vi "TEST_ASIC_MAJnADDS.vi"(0 "Instrument VISA in":T1={"AWG VISA"="generadorpulsos", "Oscilloscope  VISA "="Oscilloscope", "Integration Board IP"="172.16.7.43", "connection ID"=refnum, "report out"=refnum, "report file path"=path "C:/Documents and Settings/CTA_LAB01/Desktop/L0_Asic/L0 Asic Test "}, 1 "threshold":i32[][](array[numeric]), 2 "Serial number":string="SN002", 5 "quantity":i32=3, 7 "Cycles Burst":i32=10000, 11 "error in":errorcluster={"status"=FALSE, "code"=0, "source"="VISA Write in Test2_3a_ASIC_fast.vi->test_sum_ASIC.vi"}, 12 "channel array":i32[](array[numeric])=[0, 1, 2, 3, 4, 5, 6], 13 "Voltages comprobation":dbl[](array[numeric])=[0.05, 0.8]) -> (4 "Instrument VISA out":T1={"AWG VISA"="", "Oscilloscope  VISA "="", "Integration Board IP"="", "connection ID"=refnum, "report out"=refnum, "report file path"=path "C:/Documents and Settings/CTA_LAB01/Desktop/L0_Asic/L0 Asic Test "}, 15 "error out":errorcluster)   [LabVIEW 2009]
uses:
  <vilib>/Utility/NIReport.llb/NI_report.lvclass
  <vilib>/Utility/NIReport.llb/HTML/NI_HTML.lvclass
  <instrlib>/Agilent 81150/Agilent 81150.lvlib
  <instrlib>/Agilent 8000 Series/Agilent 8000 Series.lvlib
panel:
  out "read buffer 4":string="V amptd(f2),1.074E+00,0,1.056E+00,1.087E+00,1.0690E+00,5.5E-03,9.4E+01,+ width(f2),2.90015E-09,0,2.90015E-09,2.95960E-09,2.925838E-09,1.2702E-11,9.4E+01,V amptd(1),5.5E-02,0,4.8E-02,6.7E-02,5.55E-02,3.5E-03,9.4E+01,+ width(f1),9.99999E+37,5,9.99999E+37,9.99999E+37,9.99999E+37,9.99999E+37,9.99999E+37,Time(f1-f2),6.26722E-09,0,6.20145E-09,6.35270E-09,6.264189E-09,3.2805E-11,9.4E+01\n"
  out "report file path":path=path "C:/Documents and Settings/CTA_LAB01/Desktop/L0_Asic/L0 Asic Test "
  out "Array":i32[](array[numeric])=[2, 3, 5]
  out "points quantity":dbl=94.0
  out "ouput data array":dbl[](array[numeric])=[0.75, 42.0, 0.0, 63.0, 1.0, 1.069, 0.0055, 2.925838e-09, 1.2702e-11, 0.0555, 0.0035, 9.99999e+37, 9.99999e+37, 6.264189e-09, 3.2805e-11, 94.0]
  out "read buffer 3":string="V amptd(f2),1.074E+00,0,1.056E+00,1.087E+00,1.0690E+00,5.5E-03,9.4E+01,+ width(f2),2.90015E-09,0,2.90015E-09,2.95960E-09,2.925838E-09,1.2702E-11,9.4E+01,V amptd(1),5.5E-02,0,4.8E-02,6.7E-02,5.55E-02,3.5E-03,9.4E+01,+ width(f1),9.99999E+37,5,9.99999E+37,9.99999E+37,9.99999E+37,9.99999E+37,9.99999E+37,Time(f1-f2),6.26722E-09,0,6.20145E-09,6.35270E-09,6.264189E-09,3.2805E-11,9.4E+01\n"
  in  "Voltage":dbl[](array[numeric])=[0.05, 0.8]
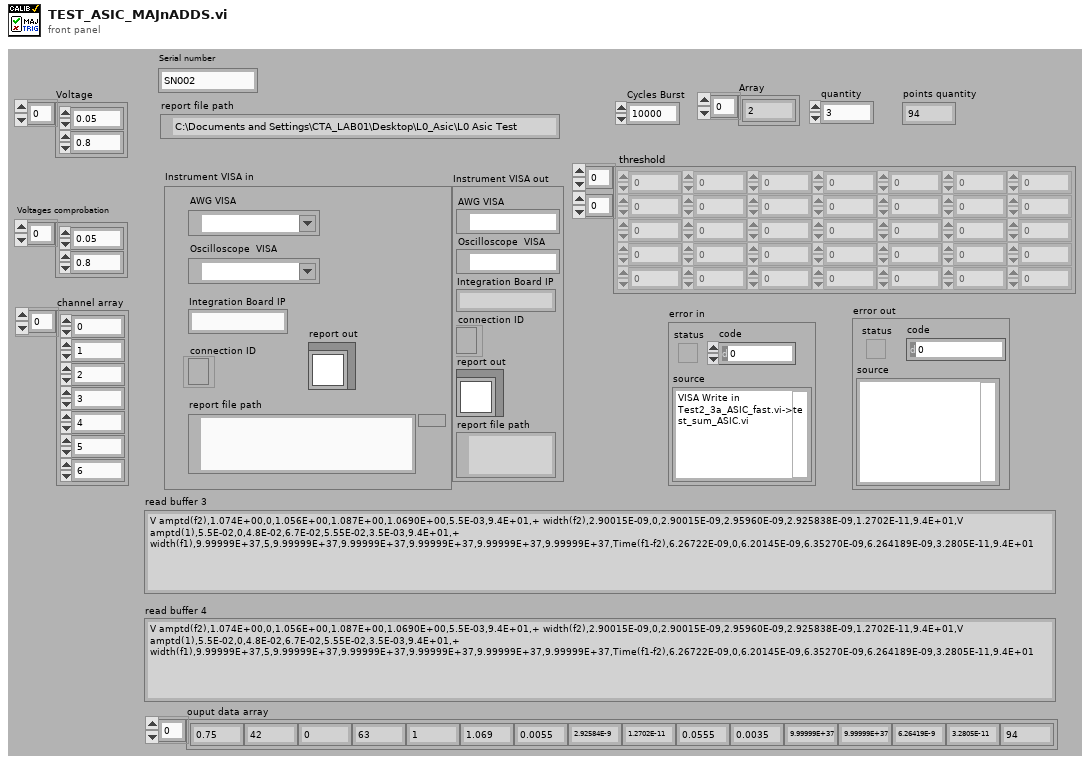
[diagram p1: front panel]
types:
  T1 = cluster{"AWG VISA":refnum<visa-resource-name>, "Oscilloscope  VISA ":refnum<visa-resource-name>, "Integration Board IP":string, "connection ID":refnum<k5>, "report out":refnum<class "NI_report.lvclass">, "report file path":path}
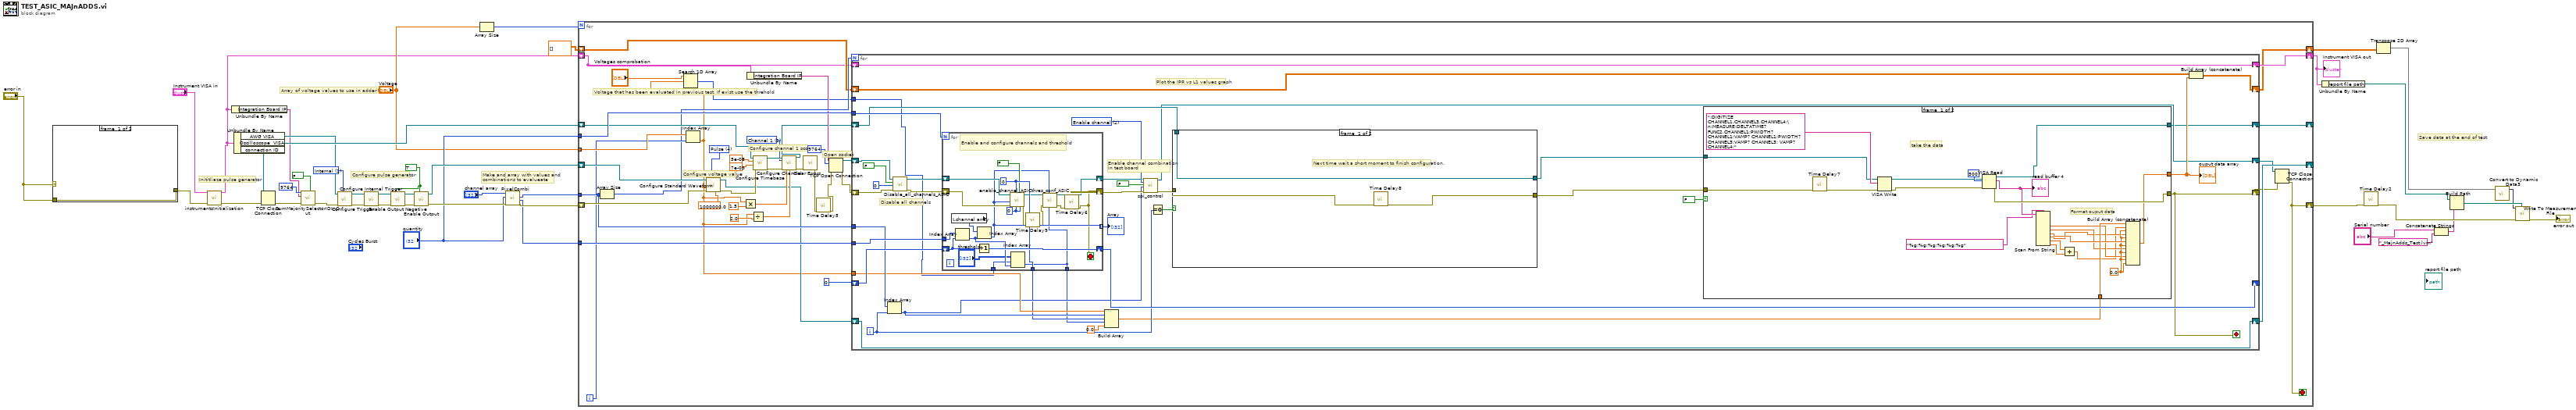
[diagram p0: block diagram]
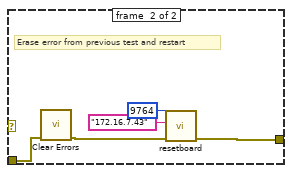
[diagram p2: hidden frame]
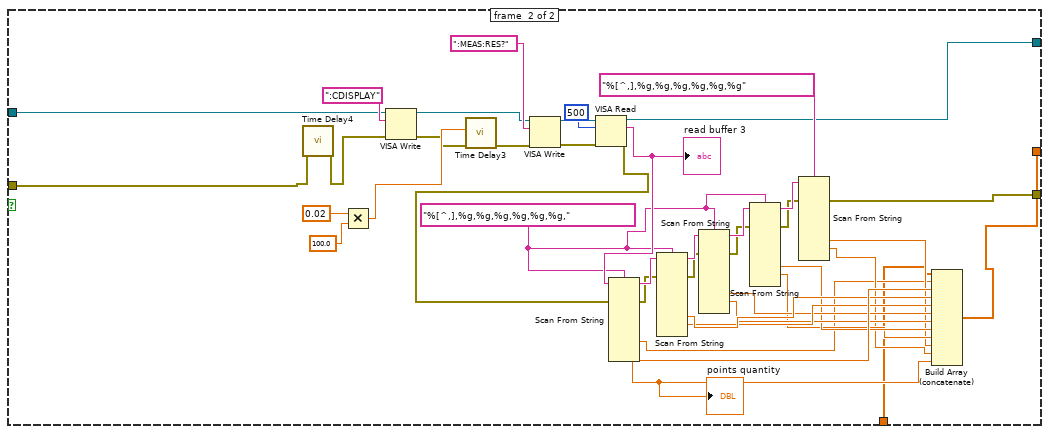
[diagram p3: hidden frame]
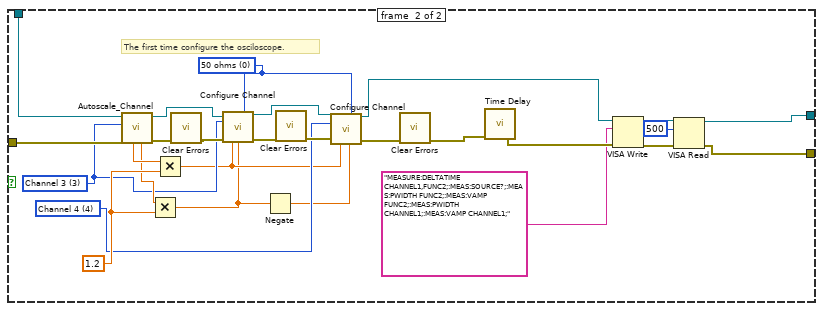
[diagram p4: hidden frame]
diagram:
  w23 = u16 1 items=["Immediate", "Internal", "External", "Software Trigger Function"] ("Trigger Source (0: Immediate)")
  w11 = TRUE ("Enable Output (T: Enable)")
  # "Save data at the end of test"
  # "Array of voltage values to use in adder test"
  # "Make and array with values and \ncombinations to evalueate"
  # "Configure pulse generator"
  # "Inititliaze pulse generator"
  n1 = case shown="Error" "error in" {
    tunnel: "error in" -> [w44 w46]
    tunnel: [w44 w49] -> w19
    frame #0 {
    }
    frame #1 {
      # "Erase error from previous test and restart"
      n2 = call <vilib>:"Clear Errors.vi"("error in (no error)"=w46) -> ("error out"=w45:errorcluster)  [unwired: 6 in]
      n3 = call "resetboard.vi"("error in (no error)"=w45, "address"="172.16.7.43", "remote port or service name"=u16 9764) -> ("error out"=w49:errorcluster)  [unwired: 7 in, 1 out]
    }
  }
  n4 = call "instrumentsInitialization.vi"("error in"=w19, "Instrument VISA in"="Instrument VISA in") -> ("error out"=w17:errorcluster, "Instrument VISA out"=w6:T1)  [unwired: 8 in]
  n5 = Unbundle By Name(w6) -> ("Integration Board IP"=w1:string)
  n6 = Unbundle By Name(w6) -> ("AWG VISA"=w26:refnum<visa-resource-name>, "Oscilloscope  VISA"=w33:refnum<visa-resource-name>, "connection ID"=w18:refnum<k5>)
  n7 = TCP Close Connection(connection ID=w18, error in (no error)=w17) -> (error out=w5:errorcluster)  [unwired: 1 in, 1 out]
  n8 = call "SumMajoritySelectorIDInOut.vi"("On Sum\nOff Majority"=FALSE ("Enable Output (T: Enable)"), "error in (no error)"=w5, "address"=w1, "remote port or service name"=u16 9764) -> ("error out"=w4:errorcluster)  [unwired: 7 in]
  n9 = call <instrlib>:"Configure Trigger.vi"("Trigger Source (0: Immediate)"=w23, "error in (no error)"=w4, "VISA resource name"=w26) -> ("error out"=w24:errorcluster, "VISA resource name out"=w25:refnum<visa-resource-name>)  [unwired: 7 in]
  n10 = call <instrlib>:"Configure Internal Trigger.vi"("error in (no error)"=w24, "VISA resource name"=w25) -> ("error out"=w13:errorcluster, "VISA resource name out"=w14:refnum<visa-resource-name>)  [unwired: 8 in]
  n11 = call <instrlib>:"Enable Output Negative.vi"("Enable Output (T: Enable)"=w11, "error in (no error)"=w13, "VISA resource name"=w14) -> ("error out"=w12:errorcluster, "VISA resource name out"=w15:refnum<visa-resource-name>)  [unwired: 7 in]
  n12 = call <instrlib>:"Enable Output.vi"("Enable Output (T: Enable)"=w11, "error in (no error)"=w12, "VISA resource name"=w15) -> ("error out"=w43:errorcluster, "VISA resource name out"=w41:refnum<visa-resource-name>)  [unwired: 7 in]
  n13 = Array Size(array="Voltage") -> (size(s)=w34:i32)
  n14 = call "PixelCombi.vi"("error in"=w43, "quantity"="quantity", "array"="channel array") -> ("error out"=w42:errorcluster, "Channels"=w40:i32[], "Combination Array"=w39:i16[])  [unwired: 6 in]
  n15 = for {
    N: w34 -> [_]
    tunnel: w40 -> [w90]
    tunnel: w39 -> [w89]
    shift-right: [w78] -> w27
    shift-left: w42 -> [w92]
    tunnel: "Voltage" -> [w88]
    tunnel: "quantity" -> [w86]
    shift-right: [w82] -> w16
    shift-left: w6 -> [w53]
    shift-right: [w81] -> w10
    shift-left: dbl[][] [] -> [w83]
    shift-right: [w79] -> _
    shift-left: w41 -> [w91]
    shift-right: [w80] -> _
    shift-left: w33 -> [w85]
    i -> [w87]
    stop <- w78 stop-if-true
    w68 = 1 items=["Channel 1"=1, "Channel 2"=2, "Channel 3"=3, "Channel 4"=4] ("Channel (1: Channel 1)")
    w77 = u16 4 items=["Sine", "Square", "Ramp Up", "Ramp Down", "Pulse", "Noise", "DC"] ("Waveform (0: Sine)")
    # "Open socket"
    # "Configure channel 1 scope"
    # "Configure voltage value"
    # "Voltage that has been evaluated in previous test. If exist use the threhold"
    n16 = Array Size(array=w89) -> (size(s)=w84:i32)
    n17 = Index Array(array=w88, index=w87) -> (element=w52:dbl)
    n18 = Search 1D Array(1D array="Voltages comprobation", element=w52) -> (index of element=w50:i32)  [unwired: 1 in]
    n19 = call <instrlib>:"Configure Standard Waveform.vi"("Frequency (1000.0 Hz)"=1000000.0, "Waveform (0: Sine)"=w77, "error in (no error)"=w92, "Amplitude (1.0 Vpp)"=w52, "VISA resource name"=w91) -> ("error out"=w74:errorcluster, "VISA resource name out"=w56:refnum<visa-resource-name>)  [unwired: 5 in]
    n20 = Multiply(x=w52, y=1.5) -> (x*y=w67:dbl)
    n21 = Unbundle By Name(w53) -> ("Integration Board IP"=w64:string)
    n22 = Divide(x=w52, y=2.0) -> (x/y=w61:dbl)
    n23 = call <instrlib>:"Configure Timebase.vi"("error in (no error)"=w74, "Position (0.0 s)"=7e-09, "Timebase (0.005 s)"=5e-08, "VISA resource name"=w85) -> ("error out"=w73:errorcluster, "VISA resource name out"=w71:refnum<visa-resource-name>)  [unwired: 6 in]
    n24 = call <instrlib>:"Configure Channel.vi"("VISA resource name"=w71, "Channel (1: Channel 1)"=w68, "error in (no error)"=w73, "Vertical Range (2.0 V)"=w67, "Vertical Offset (0.0 V)"=w61) -> ("VISA resource name out"=w60:refnum<visa-resource-name>, "error out"=w72:errorcluster)  [unwired: 9 in]
    n25 = call <vilib>:"Clear Errors.vi"("error in (no error)"=w72) -> ("error out"=w55:errorcluster)  [unwired: 6 in]
    n26 = call "Time Delay5"("error in (no error)"=w55) -> ("error out"=w54:errorcluster)  [unwired: 10 in]
    n27 = TCP Open Connection(address=w64, remote port or service name=u16 9764, error in (no error)=w54) -> (connection ID=w57:refnum<k5>, error out=w65:errorcluster)  [unwired: 2 in]
    n28 = for {
      N: w84 -> [_]
      tunnel: w89 -> [w127]
      tunnel: w90 -> [w128]
      shift-right: [w129] -> _
      shift-left: i16 0 ("element") -> [w130]
      shift-right: [w108] -> w59
      shift-left: w65 -> [w120]
      tunnel: w86 -> [w126]
      shift-right: [w121] -> w81
      shift-left: w83 -> [w122]
      shift-right: [w109] -> w58
      shift-left: w57 -> [w107]
      tunnel: w52 -> [w105]
      shift-right: [w101] -> w80
      shift-left: w60 -> [w114]
      shift-right: [w100] -> w79
      shift-left: w56 -> [w100]
      shift-right: [w95] -> w82
      shift-left: w53 -> [w95]
      tunnel: w50 -> [w93]
      i -> [w112]
      stop <- w108 stop-if-true
      w119 = u16 2 items=["Attenuation", "Clipping", "Enable channel", "Delay line", "ASIC"] ("Device")
      # "Enable channel combination \nin test board"
      # "Disable all channels"
      # "Plot the IPR vs L1 values graph"
      n29 = Index Array(array=w127, index=w112) -> (element=w104:i16)
      n30 = call "Disable_all_channels_ASIC.vi"("error in"=w120, "id_in"=0 ("Data"), "Clip_en_b"=FALSE, "connection ID"=w107) -> ("error out"=w124:errorcluster, "connection ID out"=w123:refnum<k5>)  [unwired: 5 in, 1 out]
      n31 = for {
        N: w126 -> [_]
        shift-right: [w241] -> w129
        shift-left: w130 -> [w242]
        tunnel: w128 -> [w240]
        shift-right: [w229] -> w117
        shift-left: w124 -> [w238]
        shift-right: [w232] -> w116
        shift-left: w123 -> [w237]
        tunnel: [w231] -> w106 mode=indexing
        tunnel: [w236] -> w103
        tunnel: [w230] -> w96
        tunnel: w93 -> [w226]
        stop <- w229 stop-if-true
        w234 = u32 0 ("Ib_clipVb")
        w236 = u32 0 ("Att gain")
        # "Enable and configure channels and threshold"
        n32 = local read "channel array"() -> (w239:i32[])
        n33 = Index Array(array=w240, index=w242) -> (element=w227:i32)
        n34 = Increment(x=w242) -> (x+1=w241:i16)
        n35 = Index Array(array=w239, index=w227) -> (element=w231:i32)
        n36 = call "enable_channel_ASIC.vi"("Clip_sel_b"=w234, "maj/sum"=FALSE, "Ib_clipVb"=w234, "Att gain"=w236, "error in"=w238, "Channel"=w231, "connection ID"=w237) -> ("error out"=w224:errorcluster, "connection ID out"=w233:refnum<k5>)  [unwired: 2 in, 1 out]
        n37 = Index Array(array="threshold", index (row)=w226, index (col)=w227) -> (element=w230:i32)
        n38 = call "Time Delay9"("error in (no error)"=w224) -> ("error out"=w225:errorcluster)  [unwired: 10 in]
        n39 = call "thres_conf_ASIC.vi"("threshold"=w230, "Ring"=w231, "error out 3"=w225, "connection ID"=w233) -> ("error out 2"=w228:errorcluster, "connection ID out"=w232:refnum<k5>)  [unwired: 4 in, 2 out]
        n40 = call "Time Delay6"("error in (no error)"=w228) -> ("error out"=w229:errorcluster)  [unwired: 10 in]
      }
      "Array" <- w106
      n41 = Build Array(w105, w104, w103, w96, 0.0 ("element")) -> (w102:dbl[])
      n42 = call "spi_control.vi"("connection ID"=w116, "Device"=w119, "Read/#write"=FALSE, "Data"=w104, "error out 3"=w117) -> ("connection ID out"=w109:refnum<k5>, "error out 2"=w115:errorcluster)  [unwired: 7 in, 6 out]
      n43 = Equal To 0?(x=w112) -> (x = 0?=w113:bool)
      n44 = case shown="True" w113 {
        tunnel: [w193 w202] -> w98
        tunnel: w115 -> [w194 w208]
        tunnel: w114 -> [w195 w209]
        tunnel: [w195 w211] -> w111
        frame #0 {
          # "Next time wait a short moment to finish configuration."
          n45 = call "Time Delay8"("error in (no error)"=w194) -> ("error out"=w193:errorcluster)  [unwired: 10 in]
        }
        frame #1 {
          w212 = u32 0 items=["50 ohms", "1 Mohms"] ("Input Impedance (1: 1 Mohms)")
          w200 = 3 items=["Channel 1"=1, "Channel 2"=2, "Channel 3"=3, "Channel 4"=4] ("Channel (1: Channel 1)")
          w199 = 4 items=["Channel 1"=1, "Channel 2"=2, "Channel 3"=3, "Channel 4"=4] ("Channel (1: Channel 1)")
          w205 = 1.2 ("y")
          # "The first time configure the osciloscope."
          n46 = call "Autoscale_Channel.vi"("error in"=w208, "Channel"=w200, "VISA resource name"=w209) -> ("error out"=w219:errorcluster, "VISA resource name out"=w222:refnum<visa-resource-name>, "Offset"=w201:dbl, "VerticalRange"=w216:dbl)  [unwired: 5 in]
          n47 = Multiply(x=w201, y=w205) -> (x*y=w197:dbl)
          n48 = Multiply(x=w216, y=w205) -> (x*y=w198:dbl)
          n49 = call <vilib>:"Clear Errors.vi"("error in (no error)"=w219) -> ("error out"=w220:errorcluster)  [unwired: 6 in]
          n50 = call <instrlib>:"Configure Channel.vi"("VISA resource name"=w222, "Input Impedance (1: 1 Mohms)"=w212, "Channel (1: Channel 1)"=w200, "error in (no error)"=w220, "Vertical Range (2.0 V)"=w198, "Vertical Offset (0.0 V)"=w197) -> ("VISA resource name out"=w217:refnum<visa-resource-name>, "error out"=w221:errorcluster)  [unwired: 8 in]
          n51 = Negate(x=w197) -> (-x=w196:dbl)
          n52 = call <vilib>:"Clear Errors.vi"("error in (no error)"=w221) -> ("error out"=w210:errorcluster)  [unwired: 6 in]
          n53 = call <instrlib>:"Configure Channel.vi"("VISA resource name"=w217, "Input Impedance (1: 1 Mohms)"=w212, "Channel (1: Channel 1)"=w199, "error in (no error)"=w210, "Vertical Range (2.0 V)"=w198, "Vertical Offset (0.0 V)"=w196) -> ("VISA resource name out"=w206:refnum<visa-resource-name>, "error out"=w218:errorcluster)  [unwired: 8 in]
          n54 = call <vilib>:"Clear Errors.vi"("error in (no error)"=w218) -> ("error out"=w207:errorcluster)  [unwired: 6 in]
          n55 = call "Time Delay"("error in (no error)"=w207) -> ("error out"=w204:errorcluster)  [unwired: 10 in]
          n56 = VISA Write(VISA resource name=w206, write buffer="MEASURE:DELTATIME CHANNEL1,FUNC2;:MEAS:SOURCE?;:MEAS:PWIDTH FUNC2;:MEAS:VAMP FUNC2;:MEAS:PWIDTH CHANNEL1;:MEAS:VAMP CHANNEL1;", error in (no error)=w204) -> (VISA resource name out=w215:refnum<visa-resource-name>, error out=w214:errorcluster)  [unwired: 1 out]
          n57 = VISA Read(VISA resource name=w215, byte count=u32 500, error in (no error)=w214) -> (VISA resource name out=w211:refnum<visa-resource-name>, error out=w202:errorcluster)  [unwired: 2 out]
        }
      }
      n58 = case shown="False" FALSE {
        tunnel: w111 -> [w148 w160]
        tunnel: [w143 w158] -> w110
        tunnel: [w146 w157] -> w108
        tunnel: w102 -> [w144 w155]
        tunnel: [w145 w154] -> w101
        tunnel: w98 -> [w147 w152]
        frame #0 {
          w139 = 0.0 ("output 7")
          # "Format ouput data"
          # "take the data"
          n59 = call "Time Delay7"("error in (no error)"=w147) -> ("error out"=w149:errorcluster)  [unwired: 10 in]
          n60 = VISA Write(VISA resource name=w148, write buffer=":DIGITIZE CHANNEL1,CHANNEL3,CHANNEL4;\n:MEASURE:DELTATIME? FUNC2,CHANNEL1;PWIDTH? CHANNEL1;VAMP? CHANNEL1;PWIDTH? CHANNEL3;VAMP? CHANNEL3; VAMP? CHANNEL4;", error in (no error)=w149) -> (VISA resource name out=w142:refnum<visa-resource-name>, error out=w141:errorcluster)  [unwired: 1 out]
          n61 = VISA Read(VISA resource name=w142, byte count=u32 500, error in (no error)=w141) -> (VISA resource name out=w145:refnum<visa-resource-name>, read buffer=w138:string, error out=w146:errorcluster)  [unwired: 1 out]
          "read buffer 4" <- w138
          n62 = Scan From String(format string="%g;%g;%g;%g;%g;%g", input string=w138) -> (output 1=w136:dbl, output 2=w135:dbl, output 3=w140:dbl, output 4=w134:dbl, output 5=w133:dbl, output 6=w132:dbl)  [unwired: 8 in, 3 out]
          n63 = Add(x=w133, y=w132) -> (x+y=w131:dbl)
          n64 = Build Array (concatenate)(w144, w131, w139, w134, w139, w140, w139, w135, w139, w136, w139, w139) -> (w143:dbl[])
        }
        frame #1 {
          w178 = "%[^,],%g,%g,%g,%g,%g,%g," ("format string")
          n65 = call "Time Delay4"("error in (no error)"=w152) -> ("error out"=w153:errorcluster)  [unwired: 10 in]
          n66 = Multiply(x=0.02, y=100.0) -> (x*y=w185:dbl)
          n67 = VISA Write(VISA resource name=w160, write buffer=":CDISPLAY", error in (no error)=w153) -> (VISA resource name out=w163:refnum<visa-resource-name>, error out=w161:errorcluster)  [unwired: 1 out]
          n68 = call "Time Delay3"("error in (no error)"=w161, "Delay Time (s)"=w185) -> ("error out"=w184:errorcluster)  [unwired: 9 in]
          n69 = VISA Write(VISA resource name=w163, write buffer=":MEAS:RES?", error in (no error)=w184) -> (VISA resource name out=w192:refnum<visa-resource-name>, error out=w191:errorcluster)  [unwired: 1 out]
          n70 = VISA Read(VISA resource name=w192, byte count=u32 500, error in (no error)=w191) -> (VISA resource name out=w154:refnum<visa-resource-name>, read buffer=w188:string, error out=w168:errorcluster)  [unwired: 1 out]
          "read buffer 3" <- w188
          n71 = Scan From String(format string=w178, input string=w188, error in=w168) -> (remaining string=w182:string, error out=w164:errorcluster, output 5=w156:dbl, output 6=w183:dbl, output 7=w169:dbl)  [unwired: 12 in, 1 out]
          "points quantity" <- w169
          n72 = Scan From String(format string=w178, input string=w182, error in=w164) -> (remaining string=w179:string, error out=w165:errorcluster, output 5=w176:dbl, output 6=w175:dbl)  [unwired: 13 in, 1 out]
          n73 = Scan From String(format string=w178, input string=w179, error in=w165) -> (remaining string=w180:string, error out=w166:errorcluster, output 5=w174:dbl, output 6=w173:dbl)  [unwired: 13 in, 1 out]
          n74 = Scan From String(format string=w178, input string=w180, error in=w166) -> (remaining string=w181:string, error out=w167:errorcluster, output 5=w172:dbl, output 6=w171:dbl)  [unwired: 13 in, 1 out]
          n75 = Scan From String(format string="%[^,],%g,%g,%g,%g,%g,%g", input string=w181, error in=w167) -> (error out=w157:errorcluster, output 5=w159:dbl, output 6=w170:dbl)  [unwired: 13 in, 2 out]
          n76 = Build Array (concatenate)(w155, w156, w183, w176, w175, w174, w173, w172, w171, w159, w170, w169) -> (w158:dbl[])
        }
      }
      "ouput data array" <- w110
      n77 = Build Array (concatenate)(w122, w110) -> (w121:dbl[][])
    }
    n78 = TCP Close Connection(connection ID=w58, error in (no error)=w59) -> (error out=w78:errorcluster)  [unwired: 1 in, 1 out]
  }
  "Instrument VISA out" <- w16
  n79 = Unbundle By Name(w16) -> ("report file path"=w37:path)
  n80 = call "Time Delay2"("error in (no error)"=w27) -> ("error out"=w35:errorcluster)  [unwired: 10 in]
  n81 = Transpose 2D Array(2D array=w10) -> (transposed array=w21:dbl[][])
  n82 = Concatenate Strings("Serial number", "_MajnAdds_Test.lvm" ("string")) -> (w9:string)
  n83 = Build Path(base path=w37, name or relative path=w9) -> (appended path=w36:path)
  n84 = call "Convert to Dynamic Data3"("2D Array"=w21) -> ("Dynamic Data Type"=w22:dynamicdata)  [unwired: 3 in]
  n85 = call "Write To Measurement File"("Signals"=w22, "error in (no error)"=w35, "Filename"=w36) -> ("error out"=→"error out":errorcluster)  [unwired: 14 in, 2 out]
